vi "oax_Config TIO and DSA Channels (DSA).vi"(0 "DAQ Config":T6 {"pregain" format="%.2f"; "IEPE" items=["On", "Off", "None"]; "coupling" items=["DC", "AC"]; "engineering units" items=["custom..."=0, "V"=1, "A"=21, "C"=30, "pC"=31, "s"=32, "-"=29, "Pa"=2, "N"=20, "g"=3, "m/s^2"=4, "m/s"=5, "m"=6, "mm/s"=12, "mm"=13, "micron/s"=14, "micron"=15, "in/s^2"=7, "in/s"=8, "in"=9, "mil/s"=10, "mil"=11, "rad/s^2"=16, "rad/s"=17, "rad"=18, "deg/s^2"=26, "deg/s"=27, "deg"=28, "RPM"=22, "cycle/s^2"=23, "Hz"=24, "cycle"=25, "strain"=19]; "sensor sensitivity (mV/EU)" format="%.2f"; "dB reference" format="%.1e"}, 2 "Tacho Pulse Edge":i32, 3 "Slave Slot Number":i32(ring) caption="PXI Slot Number" items=["Slot 3", "Slot 4", "Slot 5", "Slot 6", "Slot 7", "Slot 8", "Slot 9", "Slot 10", "Slot 11", "Slot 12", "Slot 13", "Slot 14", "Slot 15", "Slot 16"], 4 "DSA device type":T5 items=["4472"=0, "4474"=10, "4461"=1, "4462"=11, "4464"=12, "449x"=6, "9232"=7, "9233"=2, "9234"=3, "9229"=4, "9239"=5], 5 "error in (no error)":errorcluster, 6 "sample rate":dbl=1000.0 format="%0.2f", 7 "Counter(s)":tag="cDAQ4/_ctr0", 8 "max value":dbl=5.0 format="%0.2f", 9 "PFI line (Gate)":tag, 10 "min value":dbl=-5.0 format="%0.2f") -> (11 "channel name":string[](array[string]), 13 "channel info":T2[](array[typedef]) {"pregain" format="%.2f"; "weighting filter" items=["Linear", "A-weighting", "B-weighting", "C-weighting", "ITU-R 468-4", "Dolby", "CCITT", "C-message", "Wb", "Wc", "Wd", "We", "Wf", "Wh", "Wj", "Wk", "Wm", "AES17 20 kHz lowpass", "AES17 40 kHz lowpass", "AES17 20 kHz highpass", "AES17 40 kHz highpass"]; "dB reference" format="%^.1e"; "engineering units" items=["custom..."=0, "V"=1, "A"=21, "C"=30, "pC"=31, "s"=32, "-"=29, "Pa"=2, "N"=20, "g"=3, "m/s^2"=4, "m/s"=5, "m"=6, "mm/s"=12, "mm"=13, "micron/s"=14, "micron"=15, "in/s^2"=7, "in/s"=8, "in"=9, "mil/s"=10, "mil"=11, "rad/s^2"=16, "rad/s"=17, "rad"=18, "deg/s^2"=26, "deg/s"=27, "deg"=28, "RPM"=22, "cycle/s^2"=23, "Hz"=24, "cycle"=25, "strain"=19]; "sensor sensitivity" format="%#_5f"}, 14 "DSA task out":refnum<k21>, 15 "TIO task out":refnum<k21>, 17 "synchronization type":u16(ring) items=["by sharing sample clock", "by using reference clock"], 18 "device info":T1 {"DSA device type" items=["Custom"=0, "4472"=1, "4474"=11, "4461"=2, "4462"=12, "4464"=13, "449x"=7, "9232"=8, "9233"=3, "9234"=4, "9229"=5, "9239"=6]}, 19 "error out":errorcluster)   [LabVIEW 2017]
doc: "Configures DAQ channel properties based on the user input and starts the DAQmx task."
uses:
  <vilib>/addons/Sound and Vibration/Order Analysis/Example Support/sub VIs/OAXML_DSA DAQ Config.ctl
  <vilib>/addons/_NISVFA/_Shared subVIs/Controls/svc_Engineering Units Text Ring.ctl
  <vilib>/addons/Sound and Vibration/Order Analysis/Example Support/sub VIs/OAXML_DSA Device Type.ctl
  <vilib>/addons/_NISVFA/_Shared subVIs/Controls/svc_Channel Info.ctl
  <vilib>/addons/_NISVFA/_Shared subVIs/Controls/svc_Weighting Filter Text Ring.ctl
  <vilib>/DAQmx/configure/timing.llb/DAQmx Timing (Sample Clock).vi
  <vilib>/DAQmx/create/channels.llb/DAQmx Create Channel (CI-Count Edges).vi
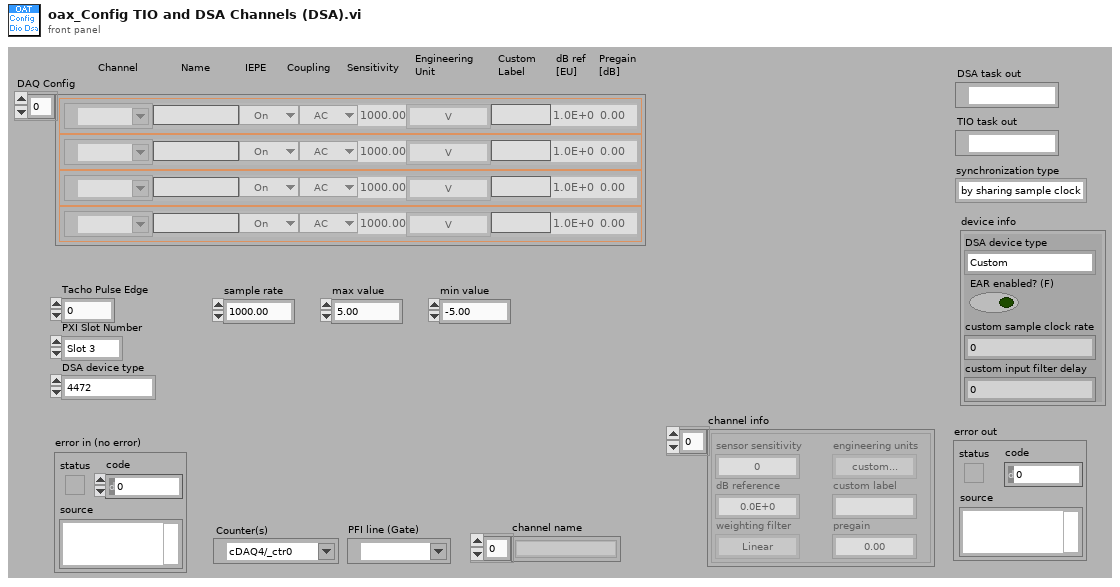
[diagram p1: front panel]
types:
  T1 = cluster{"DSA device type":u16, "EAR enabled? (F)":bool, "custom sample clock rate":dbl, "custom input filter delay":dbl}
  T2 = typedef "svc_Channel Info.ctl" = cluster{"sensor sensitivity":dbl, "engineering units":T3, "dB reference":dbl, "custom label":string, "weighting filter":T4, "pregain":dbl}
  T3 = typedef "svc_Engineering Units Text Ring.ctl" = u16
  T4 = typedef "svc_Weighting Filter Text Ring.ctl" = u16
  T5 = typedef "OAXML_DSA Device Type.ctl" = u16
  T6 = typedef "OAXML_DSA DAQ Config.ctl" = cluster{"name":string, "channel":tag, "coupling":u16, "dB reference":sgl, "sensor sensitivity (mV/EU)":dbl, "engineering units":T3, "IEPE":u16, "custom label":string, "pregain":sgl}[]
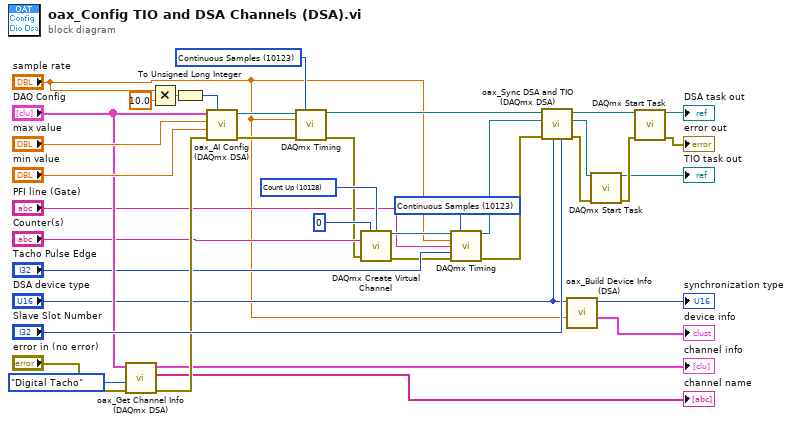
[diagram p0: block diagram]
diagram:
  w8 = 10123 items=["Finite Samples"=10178, "Continuous Samples"=10123, "Hardware Timed Single Point"=12522] ("sample mode")
  w11 = 10128 items=["Count Up"=10128, "Count Down"=10124, "Externally Controlled"=10326] ("count direction")
  w15 = 10123 items=["Finite Samples"=10178, "Continuous Samples"=10123, "Hardware Timed Single Point"=12522] ("sample mode")
  n1 = call <vilib>:"oax_Get Channel Info (DAQmx DSA).vi"("error in (no error)"="error in (no error)", "Tacho Type"=enum16{"Analog Tacho", "Digital Tacho"}."Digital Tacho", "DAQ Config"="DAQ Config") -> ("error out"=w34:errorcluster, "channel name"=→"channel name":string[], "channel info"=→"channel info":T2[])  [unwired: 3 in, 3 out]
  n2 = Multiply(x="sample rate", y=10.0) -> (x*y=w18:dbl)
  n3 = To Unsigned Long Integer(number=w18) -> (unsigned 32bit integer=w17:u32)
  n4 = call <vilib>:"oax_AI Config (DAQmx DSA).vi"("buffer size"=w17, "error in (no error)"=w34, "min value"="min value", "max value"="max value", "DAQ Config"="DAQ Config") -> ("error out"=w14:errorcluster, "task out"=w16:refnum<k21>)  [unwired: 5 in]
  n5 = call-poly <vilib>:"DAQmx Timing.vi"("task/channels in"=w16, "sample mode"=w15, "rate"="sample rate", "error in"=w14) -> ("task out"=w13:refnum<k21>, "error out"=w9:errorcluster)  [unwired: 10 in]
  n6 = call-poly <vilib>:"DAQmx Create Virtual Channel.vi"("initial count"=u32 0, "count direction"=w11, "counter"="Counter(s)", "error in"=w9) -> ("task out"=w7:refnum<k21>, "error out"=w1:errorcluster)  [unwired: 10 in]
  n7 = call-poly <vilib>:"DAQmx Timing.vi"("task/channels in"=w7, "sample mode"=w8, "rate"="sample rate", "source"="PFI line (Gate)", "active edge"="Tacho Pulse Edge", "error in"=w1) -> ("task out"=w4:refnum<k21>, "error out"=w3:errorcluster)  [unwired: 8 in]
  n8 = call <vilib>:"oax_Sync DSA and TIO (DAQmx DSA).vi"("Slave Slot Number"="Slave Slot Number", "DSA device type"="DSA device type", "error in"=w3, "TIO task in"=w4, "DSA task in"=w13) -> ("error out"=w26:errorcluster, "TIO task out"=w25:refnum<k21>, "DSA task out"=w23:refnum<k21>)  [unwired: 4 in]
  n9 = call <vilib>:"oax_Build Device Info (DSA).vi"("sample rate"="sample rate", "DSA device type"="DSA device type") -> ("device info"=→"device info":T1, "synchronization type"=→"synchronization type":u16)  [unwired: 8 in]
  n10 = call <vilib>:"DAQmx Start Task.vi"("task/channels in"=w25, "error in"=w26) -> ("task out"=→"TIO task out":refnum<k21>, "error out"=w22:errorcluster)  [unwired: 12 in]
  n11 = call <vilib>:"DAQmx Start Task.vi"("task/channels in"=w23, "error in"=w22) -> ("task out"=→"DSA task out":refnum<k21>, "error out"=→"error out":errorcluster)  [unwired: 12 in]
